vi "macro_DigSeqLogic_Delay.vi"   [LabVIEW 2019, in "Trajectory_Library.lvlib"]
uses:
  Trajectory_Library.lvlib
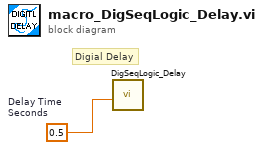
[diagram p0: block diagram]
diagram:
  w1 = 0.5  # Delay Time Seconds
  # "Digial Delay"
  n1 = call "DigSeqLogic_Delay.vi"("Delay Time"=w1) -> ()  [unwired: 9 in, 2 out]
